vi "getUserEvents.vi"(11 "Controller in":refnum<class "Controller.lvclass">) -> (2 "UserEvents":refnum<class "UserEvents.lvclass">, 3 "Controller out":refnum<class "Controller.lvclass">)   [LabVIEW 2016, in "Controller.lvclass"]
uses:
  Controller.lvclass
  UserEvents/UserEvents.lvclass
  Controller.lvclass/Controller.ctl
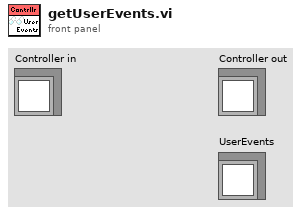
[diagram p1: front panel]
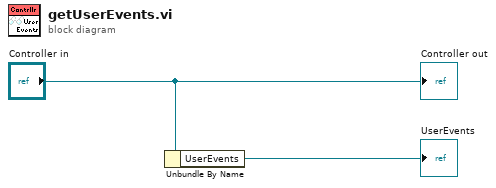
[diagram p0: block diagram]
diagram:
  n1 = Unbundle By Name("Controller in") -> ("UserEvents"=→"UserEvents":refnum<class "UserEvents.lvclass">)
  "Controller out" <- "Controller in"
